vi "Sequence Transformation To Independent Sequence for Each Channel.vi"(10 "Channel delays(s)":dbl[](array[numeric])=[0.0, 0.0, 0.0, 0.0, 0.0, 0.0, 0.0, 0.0] format="%#_6p", 11 "Array in":T3(array[cluster])) -> (2 "Time Sequence x 8 Channel":dbl[][](array[numeric]), 3 "Start Level x 8 Channel":bool[](array[boolean]))   [LabVIEW 2020]
uses:
  Labview Library/Libraries/HW_LMMR_ASG8100/LMMR ASG/Loop Config.ctl
  Labview Library/Libraries/HW_LMMR_ASG8100/LMMR ASG/Loop Code.ctl
  Labview Library/Libraries/HW_LMMR_ASG8100/LMMR ASG/Loop XControl.xctl
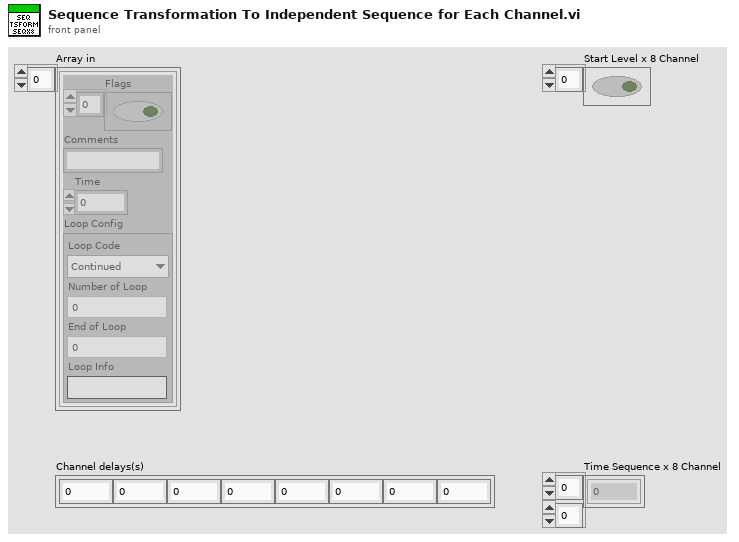
[diagram p1: front panel]
types:
  T1 = typedef "Loop XControl.xctl/Loop Config.ctl" = cluster{"Loop Code":T2, "Number of Loop":i32, "End of Loop":dbl, "Loop Info":string}
  T2 = typedef "Loop XControl.xctl/Loop Code.ctl" = enum16{"Continued", "Loop", "End Loop"}
  T3 = cluster{"Flags":bool[], "Comments":string, "Time":dbl, "Loop Config":T1}[]
  T4 = cluster{"Flags":bool[], "Comments":string, "Time":dbl, "Loop Config":T1}
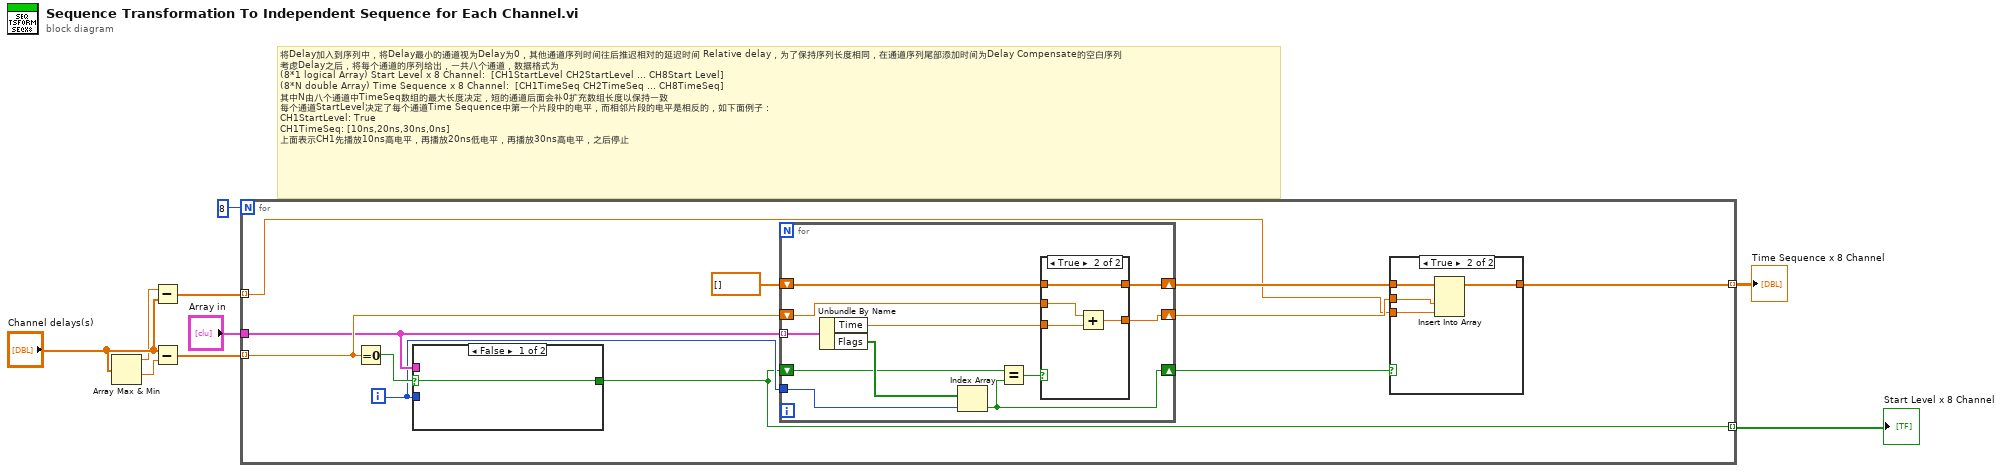
[diagram p0: block diagram]
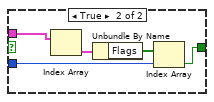
[diagram p2: hidden frame]
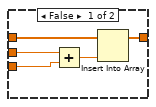
[diagram p3: hidden frame]
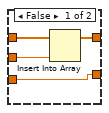
[diagram p4: hidden frame]
diagram:
  # "将Delay加入到序列中，将Delay最小的通道视为Delay为0，其他通道序列时间往后推迟相对的延迟时间 Relative delay，为了保持序列长度相同，在通道序列尾部添加时间为Delay Compensate的空白序列\n考虑Delay之后，将每个通道的序列给出，一共八个通道，数据格式为\n(8*1 logical Array)\tStart Level x 8 Channel: \t[CH1StartLevel CH2StartLevel ... CH8Start Level]\n(8*N double Array)\tTime Sequence x 8 Channel: \t[CH1TimeSeq CH2TimeSeq ... CH8TimeSeq]\n其中N由八个通道中TimeSeq数组的最大长度决定，短的通道后面会补0扩充数组长度以保持一致\n每个通道StartLevel决定了每个通道Time Sequence中第一个片段中的电平，而相邻片段的电平是相反的，如下面例子：\nCH1StartLevel: True\nCH1TimeSeq: [10ns,20ns,30ns,0ns]\n上面表示CH1先播放10ns高电平，再播放20ns低电平，再播放30ns高电平，之后停止"
  n1 = Array Max & Min(array="Channel delays(s)") -> (max value=w5:dbl, min value=w1:dbl)  [unwired: 2 out]
  n2 = Subtract(x=w5, y="Channel delays(s)") -> (x-y=w7:dbl[])
  n3 = Subtract(x="Channel delays(s)", y=w1) -> (x-y=w4:dbl[])
  n4 = for {
    N: 8 -> [_]
    tunnel: "Array in" -> [w12]
    tunnel: w4 -> [w14] mode=indexing
    tunnel: [w17] -> w8 mode=indexing
    tunnel: w7 -> [w15] mode=indexing
    tunnel: [w10] -> w9 mode=indexing
    i -> [w11]
    n5 = Equal To 0?(x=w14) -> (x = 0?=w13:bool)
    n6 = case shown="False" w13 {
      selector: w13 -> [w21 _]
      tunnel: w12 -> [_ w26]
      tunnel: w11 -> [_ w23]
      tunnel: [w21 w22] -> w10
      frame False {
      }
      frame True {
        n7 = Index Array(array=w26) -> (element=w25:T4)  [unwired: 1 in]
        n8 = Unbundle By Name(w25) -> ("Flags"=w24:bool[])
        n9 = Index Array(array=w24, index=w23) -> (element=w22:bool)
      }
    }
    n10 = for {
      tunnel: w12 -> [w46] mode=indexing
      shift-right: [w36] -> w19
      shift-left: w10 -> [w44]
      shift-right: [w41] -> w16
      shift-left: w14 -> [w40]
      tunnel: w11 -> [w39]
      shift-right: [w38] -> w18
      shift-left: dbl[] [] -> [w37]
      n11 = Unbundle By Name(w46) -> ("Time"=w42:dbl, "Flags"=w45:bool[])
      n12 = Index Array(array=w45, index=w39) -> (element=w36:bool)
      n13 = Equal?(x=w44, y=w36) -> (x = y?=w43:bool)
      n14 = case shown="True" w43 {
        tunnel: w42 -> [w49 w53]
        tunnel: [w49 w52] -> w41
        tunnel: w40 -> [w50 w54]
        tunnel: [w48 w51] -> w38
        tunnel: w37 -> [w47 w51]
        frame False {
          n15 = Insert Into Array(array=w47, new element=w50) -> (w48:dbl[])  [unwired: 1 in]
        }
        frame True {
          n16 = Add(x=w54, y=w53) -> (x+y=w52:dbl)
        }
      }
    }
    n17 = case shown="True" w19 {
      tunnel: w15 -> [w28 w32]
      tunnel: [w31 w35] -> w17
      tunnel: w18 -> [w30 w34]
      tunnel: w16 -> [w29 w33]
      frame False {
        n18 = Add(x=w29, y=w28) -> (x+y=w27:dbl)
        n19 = Insert Into Array(array=w30, new element=w27) -> (w31:dbl[])  [unwired: 1 in]
      }
      frame True {
        n20 = Insert Into Array(array=w34, new element #1=w33, new element #2=w32) -> (w35:dbl[])  [unwired: 1 in]
      }
    }
  }
  "Start Level x 8 Channel" <- w9
  "Time Sequence x 8 Channel" <- w8
